vi "Spreadsheet Storage (OpenWriteClose).vi"() -> ()   [LabVIEW 2015]
panel:
  in  "Waveform Parameters":T1
  in  "Digitizing Parameters":T2
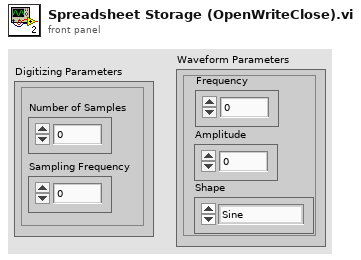
[diagram p1: front panel]
types:
  T1 = cluster{"Frequency":dbl, "Amplitude":dbl, "Shape":enum16{"Sine", "Cosine", "DC Level", "Square", "User-Defined"}}
  T2 = cluster{"Number of Samples":i32, "Sampling Frequency":dbl}
  T3 = enum16{"open", "replace", "create", "open or create", "replace or create", "replace or create with confirmation"}
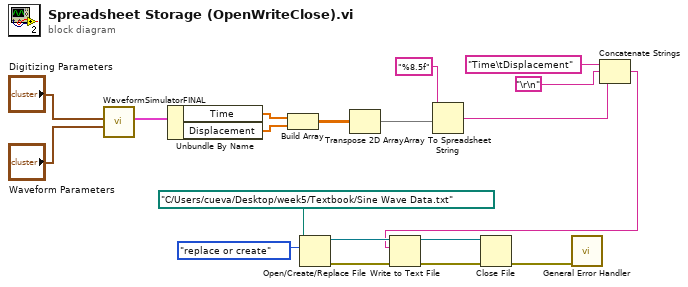
[diagram p0: block diagram]
diagram:
  n1 = call "WaveformSimulatorFINAL.vi"("Waveform Parameters"="Waveform Parameters", "Digitizing Parameters"="Digitizing Parameters") -> ("Waveform Output"=w17:cluster{"Time":dbl[], "Displacement":dbl[]})  [unwired: 9 in]
  n2 = Unbundle By Name(w17) -> ("Time"=w16:dbl[], "Displacement"=w15:dbl[])
  n3 = Build Array(w16, w15) -> (w8:dbl[][])
  n4 = Open/Create/Replace File(file path (use dialog)=path "C:/Users/cueva/Desktop/week5/Textbook/Sine Wave Data.txt" ("file path (dialog if empty)"), operation (0:open)=T3."replace or create") -> (refnum out=w5:refnum<file>, error out=w12:errorcluster)  [unwired: 4 in, 1 out]
  n5 = Transpose 2D Array(2D array=w8) -> (transposed array=w7:dbl[][])
  n6 = Array To Spreadsheet String(array=w7, 3:"%8.5f" ("format (%.3f)")) -> (spreadsheet string=w4:string)  [unwired: 1 in]
  n7 = Concatenate Strings("Time\tDisplacement" ("string"), "\r\n", w4) -> (w3:string)
  n8 = Write to Text File(file (use dialog)=w5, text=w3, error in=w12) -> (refnum out=w13:refnum<file>, error out=w11:errorcluster)  [unwired: 1 in, 1 out]
  n9 = Close File(refnum=w13, error in=w11) -> (error out=w10:errorcluster)  [unwired: 1 out]
  n10 = call <vilib>:"General Error Handler.vi"("error in (no error)"=w10) -> ()  [unwired: 10 in, 5 out]
